vi "RI_Data to dB_Data.vi"(0 "Port Type":u16(ring), 1 "Sxx_R":dbl[][](array[numeric]), 2 "Sxx_I":dbl[][](array[numeric]), 4 "S-Parameter Name":T1(ring)) -> (14 "Single S-parameters Data":dbl[][](array[numeric]), 15 "Diff S-parameters Data":dbl[][](array[numeric]))   [LabVIEW 2011]
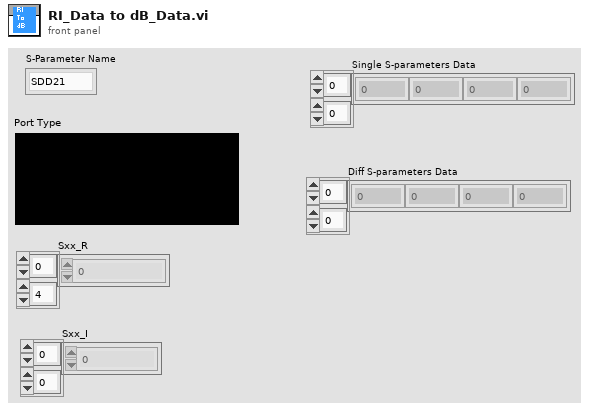
[diagram p1: front panel]
types:
  T1 = enum16{"SDD21", "SDD12", "SDD11", "SDD22", "SCD21", "SCD12", "SCD22", "SCD11", "SDC11", "SDC22", "SDC12", "SDC21", "SCC11", "SCC22", "SCC12", "SCC21"}
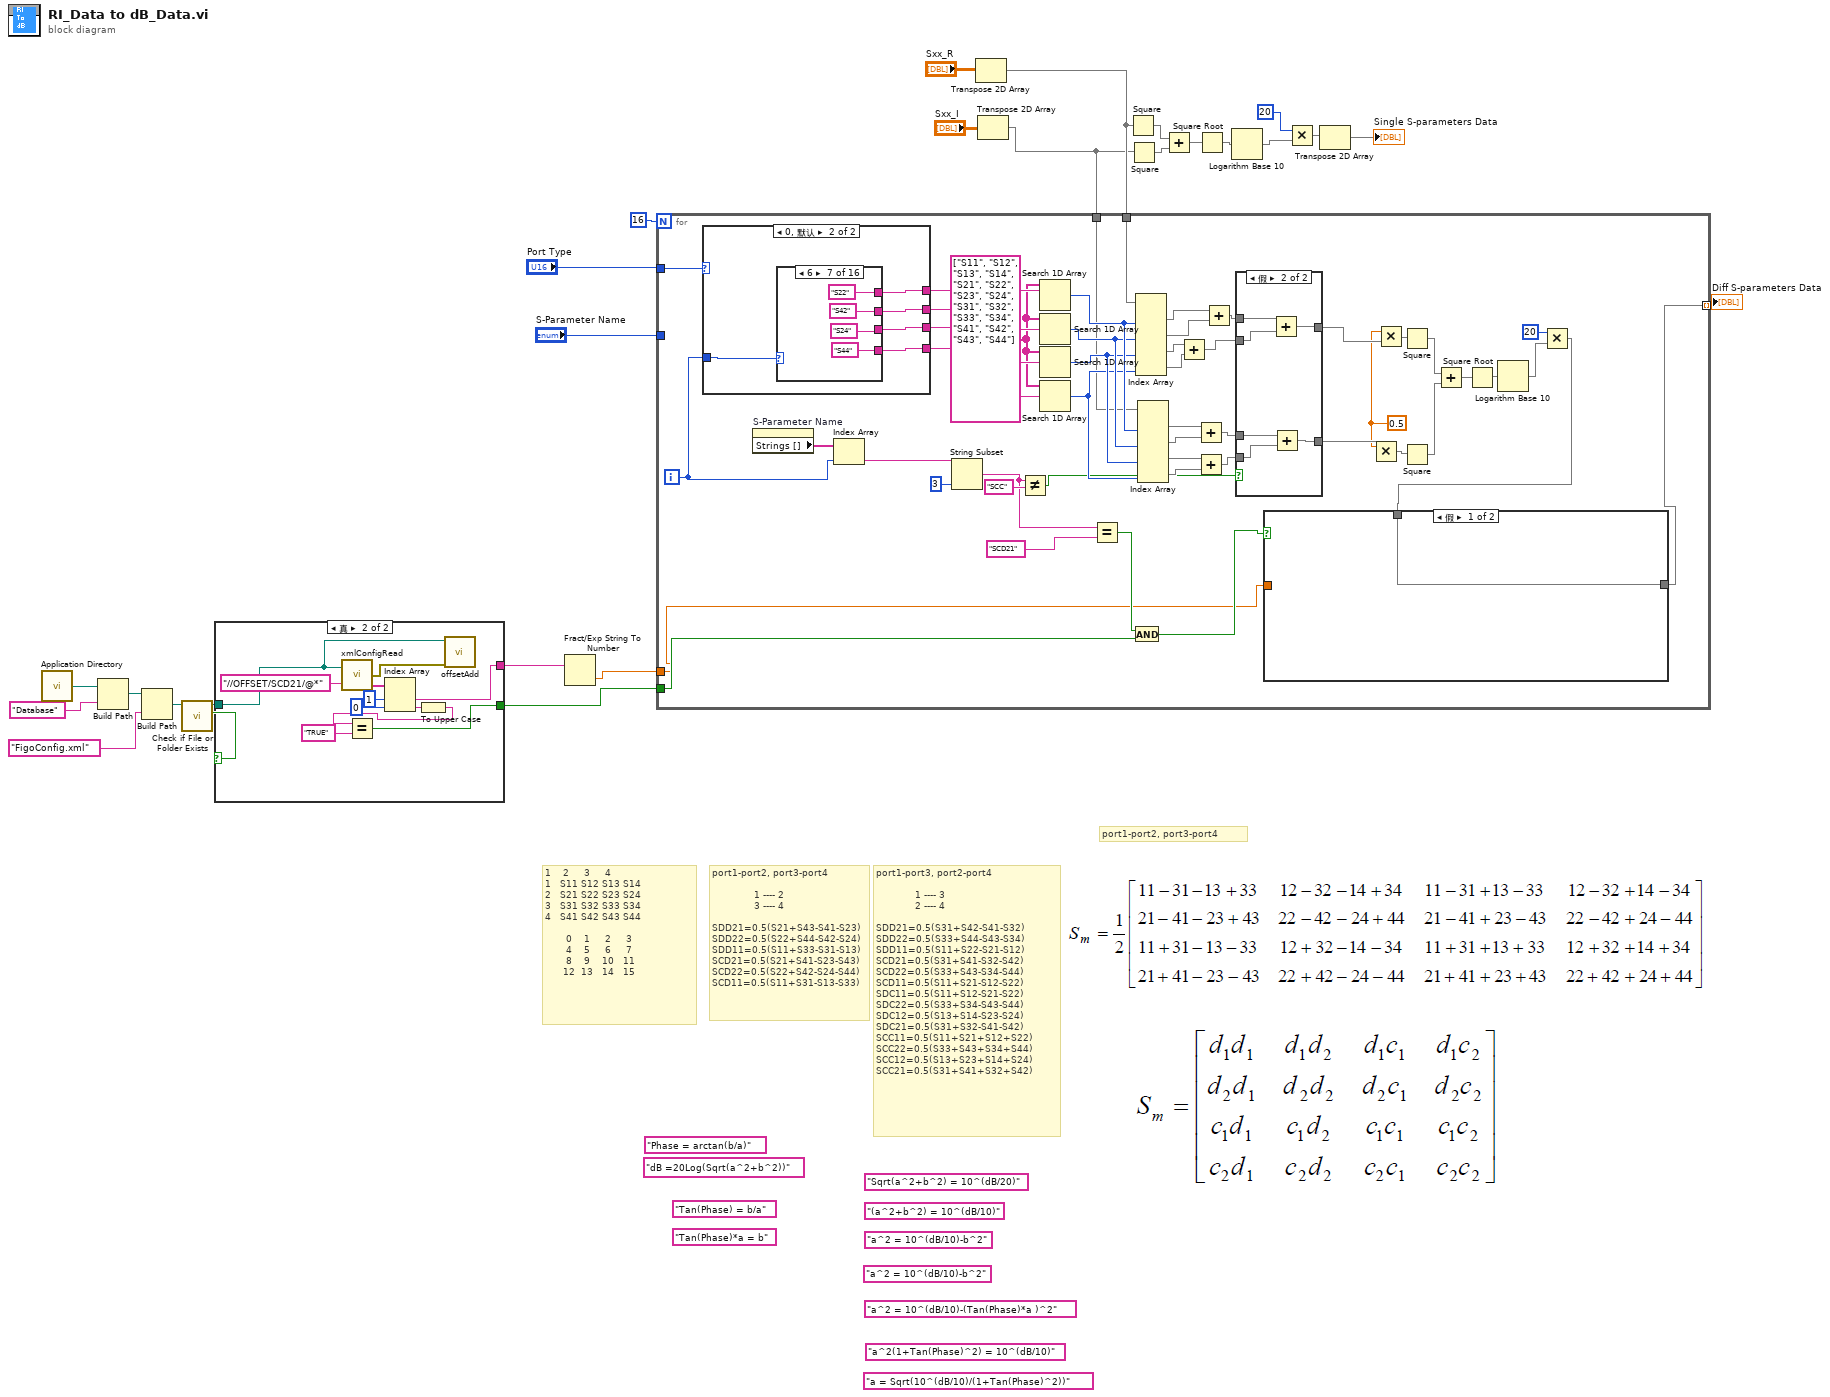
[diagram p0: block diagram]
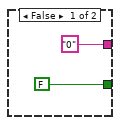
[diagram p2: hidden frame]
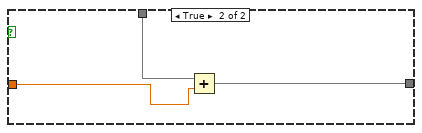
[diagram p3: hidden frame]
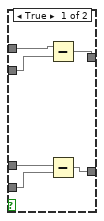
[diagram p4: hidden frame]
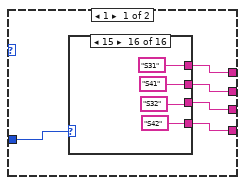
[diagram p5: hidden frame]
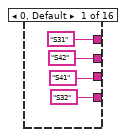
[diagram p6: hidden frame]
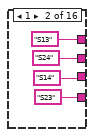
[diagram p7: hidden frame]
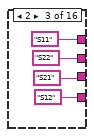
[diagram p8: hidden frame]
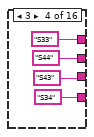
[diagram p9: hidden frame]
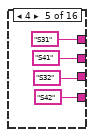
[diagram p10: hidden frame]
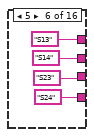
[diagram p11: hidden frame]
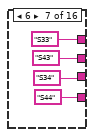
[diagram p12: hidden frame]
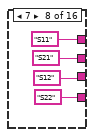
[diagram p13: hidden frame]
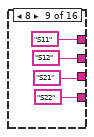
[diagram p14: hidden frame]
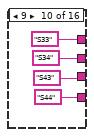
[diagram p15: hidden frame]
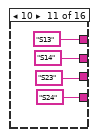
[diagram p16: hidden frame]
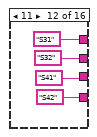
[diagram p17: hidden frame]
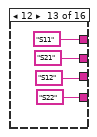
[diagram p18: hidden frame]
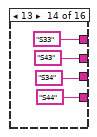
[diagram p19: hidden frame]
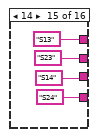
[diagram p20: hidden frame]
diagram:
  (unwired) "a = Sqrt(10^(dB/10)/(1+Tan(Phase)^2))"
  (unwired) "a^2(1+Tan(Phase)^2) = 10^(dB/10)"
  (unwired) "a^2 = 10^(dB/10)-(Tan(Phase)*a )^2"
  (unwired) "Tan(Phase)*a = b"
  (unwired) "a^2 = 10^(dB/10)-b^2"
  (unwired) "a^2 = 10^(dB/10)-b^2"
  (unwired) "(a^2+b^2) = 10^(dB/10)"
  (unwired) "Sqrt(a^2+b^2) = 10^(dB/20)"
  (unwired) "Tan(Phase) = b/a"
  (unwired) "dB =20Log(Sqrt(a^2+b^2))"
  (unwired) "Phase = arctan(b/a)"
  # "port1-port2, port3-port4"
  # "port1-port3, port2-port4\n \n             1 ---- 3\n             2 ---- 4\n\nSDD21=0.5(S31+S42-S41-S32)\nSDD22=0.5(S33+S44-S43-S34)\nSDD11=0.5(S11+S22-S21-S12)\nSCD21=0.5(S31+S41-S32-S42)\nSCD22=0.5(S33+S43-S34-S44)\nSCD11=0.5(S11+S21-S12-S22)\nSDC11=0.5(S11+S12-S21-S22)\nSDC22=0.5(S33+S34-S43-S44)\nSDC12=0.5(S13+S14-S23-S24)\nSDC21=0.5(S31+S32-S41-S42)\nSCC11=0.5(S11+S21+S12+S22)\nSCC22=0.5(S33+S43+S34+S44)\nSCC12=0.5(S13+S23+S14+S24)\nSCC21=0.5(S31+S41+S32+S42)"
  # "port1-port2, port3-port4\n\n              1 ---- 2\n              3 ---- 4\n\nSDD21=0.5(S21+S43-S41-S23)\nSDD22=0.5(S22+S44-S42-S24)\nSDD11=0.5(S11+S33-S31-S13)\nSCD21=0.5(S21+S41-S23-S43)\nSCD22=0.5(S22+S42-S24-S44)\nSCD11=0.5(S11+S31-S13-S33)"
  # "1    2     3     4\n1   S11 S12 S13 S14 \n2   S21 S22 S23 S24\n3   S31 S32 S33 S34\n4   S41 S42 S43 S44\n\n       0    1     2     3\n       4    5     6     7\n       8    9    10   11\n      12  13   14   15"
  n1 = call <vilib>:"Application Directory.vi"() -> ("Application Directory"=w8:path)
  n2 = Build Path(base path=w8, name or relative path="Database" ("名称或相对路径")) -> (appended path=w10:path)
  n3 = Build Path(base path=w10, name or relative path="FigoConfig.xml" ("名称或相对路径")) -> (appended path=w7:path)
  n4 = call <vilib>:"Check if File or Folder Exists.vi"("path"=w7) -> ("file or folder exists?"=w6:bool, "dup path"=w5:path)  [unwired: 8 in, 1 out]
  n5 = case shown="真" w6 {
    tunnel: w5 -> [_ w33]
    tunnel: [FALSE w35] -> w1
    tunnel: ["0" ("node text") w34] -> w3
    frame False {
    }
    frame True {
      n6 = call "xmlConfigRead.vi"("path to XML document"=w33, "XPath expression"="//OFFSET/SCD21/@*") -> ("error out"=w32:errorcluster, "OutParaArray"=w31:string[])  [unwired: 1 out]
      n7 = Index Array(array=w31, index #1=1 ("索引"), index #2=0 ("索引")) -> (element #1=w34:string, element #2=w38:string)
      n8 = To Upper Case(1:w38) -> (0:w37:string)
      n9 = Equal?(x=w37, y="TRUE") -> (x = y?=w35:bool)
      n10 = call "offsetAdd.vi"("error in (no error)"=w32, "xmlConfigPath"=w33) -> ()  [unwired: 9 in, 1 out]
    }
  }
  n11 = Fract/Exp String To Number(string=w3) -> (number=w2:dbl)  [unwired: 3 in, 1 out]
  n12 = Transpose 2D Array(2D array="Sxx_R") -> (transposed array=w16:dbl[][])
  n13 = Transpose 2D Array(2D array="Sxx_I") -> (transposed array=w15:dbl[][])
  n14 = for {
    N: 16 -> [_]
    tunnel: "S-Parameter Name" -> [_]
    tunnel: "Port Type" -> [w64]
    tunnel: w16 -> [w63]
    tunnel: w15 -> [w62]
    tunnel: [w40] -> w13 mode=indexing
    tunnel: w2 -> [w42]
    tunnel: w1 -> [w45]
    i -> [w60]
    w48 = 0.5
    w84 = string[] ["S11", "S12", "S13", "S14", "S21", "S22", "S23", "S24", "S31", "S32", "S33", "S34", "S41", "S42", "S43", "S44"] ("子数组")
    n15 = case shown="0, 默认" w64 {
      tunnel: [w109 w178] -> w88
      tunnel: [w108 w177] -> w87
      tunnel: [w107 w176] -> w86
      tunnel: [w106 w175] -> w85
      tunnel: w60 -> [w105 w174]
      frame 1 {
        n16 = case shown="15" w105 {
          tunnel: ["S31" "S13" "S11" "S33" "S31" "S13" "S33" "S11" "S11" "S33" "S13" "S31" "S11" "S33" "S13" "S31"] -> w109
          tunnel: ["S42" "S24" "S22" "S44" "S41" "S14" "S43" "S21" "S12" "S34" "S14" "S32" "S21" "S43" "S23" "S41"] -> w108
          tunnel: ["S41" "S14" "S21" "S43" "S32" "S23" "S34" "S12" "S21" "S43" "S23" "S41" "S12" "S34" "S14" "S32"] -> w107
          tunnel: ["S32" "S23" "S12" "S34" "S42" "S24" "S44" "S22" "S22" "S44" "S24" "S42" "S22" "S44" "S24" "S42"] -> w106
          frame 0, Default {
          }
          frame 1 {
          }
          frame 2 {
          }
          frame 3 {
          }
          frame 4 {
          }
          frame 5 {
          }
          frame 6 {
          }
          frame 7 {
          }
          frame 8 {
          }
          frame 9 {
          }
          frame 10 {
          }
          frame 11 {
          }
          frame 12 {
          }
          frame 13 {
          }
          frame 14 {
          }
          frame 15 {
          }
        }
      }
      frame 0, Default {
        n17 = case shown="6" w174 {
          tunnel: ["S21" "S12" "S11" "S22" "S21" "S12" "S22" "S11" "S11" "S22" "S12" "S21" "S11" "S22" "S12" "S21"] -> w178
          tunnel: ["S43" "S34" "S33" "S44" "S41" "S32" "S42" "S31" "S13" "S24" "S14" "S23" "S31" "S42" "S32" "S41"] -> w177
          tunnel: ["S41" "S14" "S31" "S42" "S23" "S14" "S24" "S13" "S31" "S42" "S32" "S41" "S13" "S24" "S14" "S23"] -> w176
          tunnel: ["S23" "S23" "S13" "S24" "S43" "S34" "S44" "S33" "S33" "S44" "S34" "S43" "S33" "S44" "S34" "S43"] -> w175
          frame 0, Default {
          }
          frame 1 {
          }
          frame 2 {
          }
          frame 3 {
          }
          frame 4 {
          }
          frame 5 {
          }
          frame 6 {
          }
          frame 7 {
          }
          frame 8 {
          }
          frame 9 {
          }
          frame 10 {
          }
          frame 11 {
          }
          frame 12 {
          }
          frame 13 {
          }
          frame 14 {
          }
          frame 15 {
          }
        }
      }
    }
    n18 = property on="S-Parameter Name" class="Enum (严格)"() -> ("Strings []"=w61:string[])  [unwired: 2 in, 2 out]
    n19 = Index Array(array=w61, index=w60) -> (element=w59:string)
    n20 = String Subset(string=w59, length (rest)=3 ("长度（剩余）")) -> (substring=w47:string)  [unwired: 1 in]
    n21 = Not Equal?(x=w47, y="SCC") -> (x != y?=w69:bool)
    n22 = Search 1D Array(1D array=w84, element=w88) -> (index of element=w83:i32)  [unwired: 1 in]
    n23 = Search 1D Array(1D array=w84, element=w87) -> (index of element=w82:i32)  [unwired: 1 in]
    n24 = Search 1D Array(1D array=w84, element=w86) -> (index of element=w81:i32)  [unwired: 1 in]
    n25 = Search 1D Array(1D array=w84, element=w85) -> (index of element=w80:i32)  [unwired: 1 in]
    n26 = Equal?(x=w47, y="SCD21") -> (x = y?=w44:bool)
    n27 = And(x=w44, y=w45) -> (x .and. y?=w43:bool)
    n28 = Index Array(array=w63, index (col) #1=w83, index (col) #2=w82, index (col) #3=w81, index (col) #4=w80) -> (element #1=w79:dbl[], element #2=w78:dbl[], element #3=w77:dbl[], element #4=w76:dbl[])  [unwired: 4 in]
    n29 = Index Array(array=w62, index (col) #1=w83, index (col) #2=w82, index (col) #3=w81, index (col) #4=w80) -> (element #1=w75:dbl[], element #2=w74:dbl[], element #3=w73:dbl[], element #4=w72:dbl[])  [unwired: 4 in]
    n30 = Add(x=w77, y=w76) -> (x+y=w65:dbl[])
    n31 = Add(x=w75, y=w74) -> (x+y=w68:dbl[])
    n32 = Add(x=w73, y=w72) -> (x+y=w67:dbl[])
    n33 = Add(x=w79, y=w78) -> (x+y=w66:dbl[])
    n34 = case shown="假" w69 {
      tunnel: [w98 w104] -> w57
      tunnel: [w97 w103] -> w58
      tunnel: w68 -> [w96 w102]
      tunnel: w67 -> [w95 w101]
      tunnel: w66 -> [w94 w100]
      tunnel: w65 -> [w93 w99]
      frame True {
        n35 = Subtract(x=w94, y=w93) -> (x-y=w98:dbl[])
        n36 = Subtract(x=w96, y=w95) -> (x-y=w97:dbl[])
      }
      frame False {
        n37 = Add(x=w100, y=w99) -> (x+y=w104:dbl[])
        n38 = Add(x=w102, y=w101) -> (x+y=w103:dbl[])
      }
    }
    n39 = Multiply(x=w48, y=w58) -> (x*y=w51:dbl[])
    n40 = Multiply(x=w48, y=w57) -> (x*y=w50:dbl[])
    n41 = Square(x=w50) -> (x^2=w55:dbl[])
    n42 = Square(x=w51) -> (x^2=w54:dbl[])
    n43 = Add(x=w55, y=w54) -> (x+y=w53:dbl[])
    n44 = Square Root(x=w53) -> (sqrt(x)=w52:dbl[])
    n45 = Logarithm Base 10(1:w52) -> (0:w49:dbl[])
    n46 = Multiply(x=20, y=w49) -> (x*y=w41:dbl[])
    n47 = case shown="假" w43 {
      tunnel: w42 -> [_ w91]
      tunnel: w41 -> [w89 w92]
      tunnel: [w89 w90] -> w40
      frame False {
      }
      frame True {
        n48 = Add(x=w92, y=w91) -> (x+y=w90:dbl[])
      }
    }
  }
  "Diff S-parameters Data" <- w13
  n49 = Square(x=w16) -> (x^2=w23:dbl[][])
  n50 = Square(x=w15) -> (x^2=w22:dbl[][])
  n51 = Add(x=w23, y=w22) -> (x+y=w18:dbl[][])
  n52 = Square Root(x=w18) -> (sqrt(x)=w20:dbl[][])
  n53 = Logarithm Base 10(1:w20) -> (0:w21:dbl[][])
  n54 = Multiply(x=20, y=w21) -> (x*y=w17:dbl[][])
  n55 = Transpose 2D Array(2D array=w17) -> (transposed array=→"Single S-parameters Data":dbl[][])
